vi "UI.vi"() -> ()   [LabVIEW 2024]
uses:
  Cryptography-main/Cryptography-main/src/MD5/MD5.lvlib
  Cryptography-main/Cryptography-main/src/SHA-1/SHA-1.lvlib
panel:
  in  "Text":string
  out "Execution Time":dbl
  out "Result":string
  in  "Run":bool
  in  "File Input":path
  in  "Select a Tool":i32(listbox)
  # "Forensics and cryptography Lab"
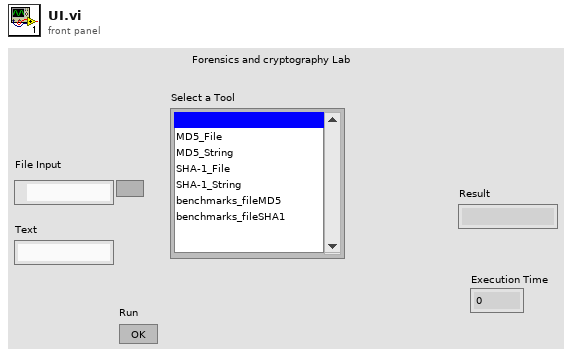
[diagram p1: front panel]
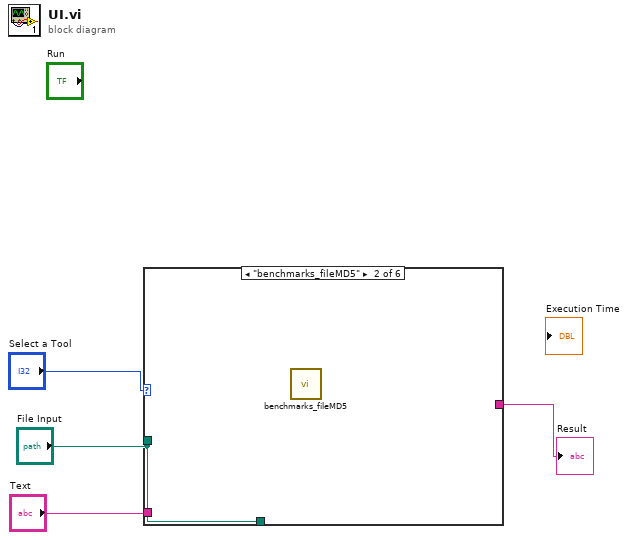
[diagram p0: block diagram]
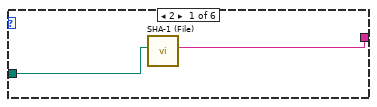
[diagram p2: hidden frame]
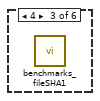
[diagram p3: hidden frame]
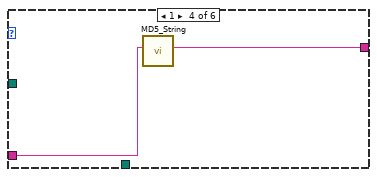
[diagram p4: hidden frame]
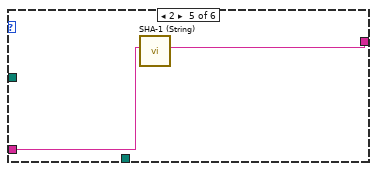
[diagram p5: hidden frame]
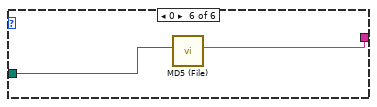
[diagram p6: hidden frame]
diagram:
  n1 = case shown="\"benchmarks_fileMD5\"" "Select a Tool" {
    tunnel: "File Input" -> [_ _ _ _ _ _]
    tunnel: [w5 _ _ _ w10 w11] -> _
    tunnel: "File Input" -> [w6 _ _ _ _ w12]
    tunnel: "Text" -> [_ _ _ w8 w9 _]
    tunnel: [_ _ _ w7 _ _] -> w1
    frame 2 {
      n2 = call "SHA-1 (File).vi"("filepath"=w6) -> ("SHA-1 hash"=w5:string)  [unwired: 10 in]
    }
    frame 3 {
      n3 = call "benchmarks_fileMD5.vi"() -> ()  [unwired: 12 in]
    }
    frame 4 {
      n4 = call "benchmarks_fileSHA1.vi"() -> ()  [unwired: 12 in]
    }
    frame 1 {
      n5 = call "MD5_String.vi"("message"=w8) -> ("MD5 hash"=w7:string)  [unwired: 10 in]
    }
    frame 2 {
      n6 = call "SHA-1 (String).vi"("message"=w9) -> ("SHA-1 hash"=w10:string)  [unwired: 10 in]
    }
    frame 0 {
      n7 = call "MD5 (File).vi"("filepath"=w12) -> ("MD5 hash"=w11:string)  [unwired: 10 in]
    }
  }
  "Result" <- w1
